vi "Programa Principal.vi"() -> ()   [LabVIEW 2017]
uses:
  <vilib>/Instr/_visa.llb/Select Event Type.ctl
  <vilib>/addons/_office/_exclsub.llb/font.ctl
  <vilib>/Utility/NIReport.llb/Append Report Text (str wrap).vi
  <vilib>/Utility/NIReport.llb/NI_report.lvclass
  <vilib>/addons/_office/NI_ReportGenerationToolkit.lvlib
  <vilib>/Utility/NIReport.llb/Word/NI_Word.lvclass
panel:
  in  "report file path":path
  in  "Guardar":bool
  in  "COMENTARIO":string
  in  "Prac5":bool
  in  "stop 2":bool
  out "Byte recibido":u16
  out "Byte enviado":u32
  out "Datos recibidos":u8[](array[numeric])
  in  "VISA resource name":refnum<visa-resource-name>
  out "Grafica":dbl(graph)
  out "O4":bool
  out "O5":bool
  out "O6":bool
  out "O7":bool
  out "O8":bool
  in  "S4":bool
  in  "S5":bool
  in  "S6":bool
  in  "S7":bool
  in  "S8":bool
  out "Tiempo de Muestreo (ms)":dbl format="%#_5g"
  in  "Semi. Aut.":bool
  in  "Aut.":bool
  out "Manual 2":bool caption="Manual"
  in  "Manual":bool
  out "Automatico 2":bool
  out "Sem.Aut.":bool
  out "Emergencia 2":bool caption="Manual"
  in  "Emergencia":bool
  in  "stop":bool
  in  "Prac4":bool
  in  "Base de Datos":bool
  # "TABLERO DE COMUNICACION"
  # "TABLERO DE CONTRLOL"
  # "ON"
  # "OFF"
  # "LABORATORIO DE MATERIALES"
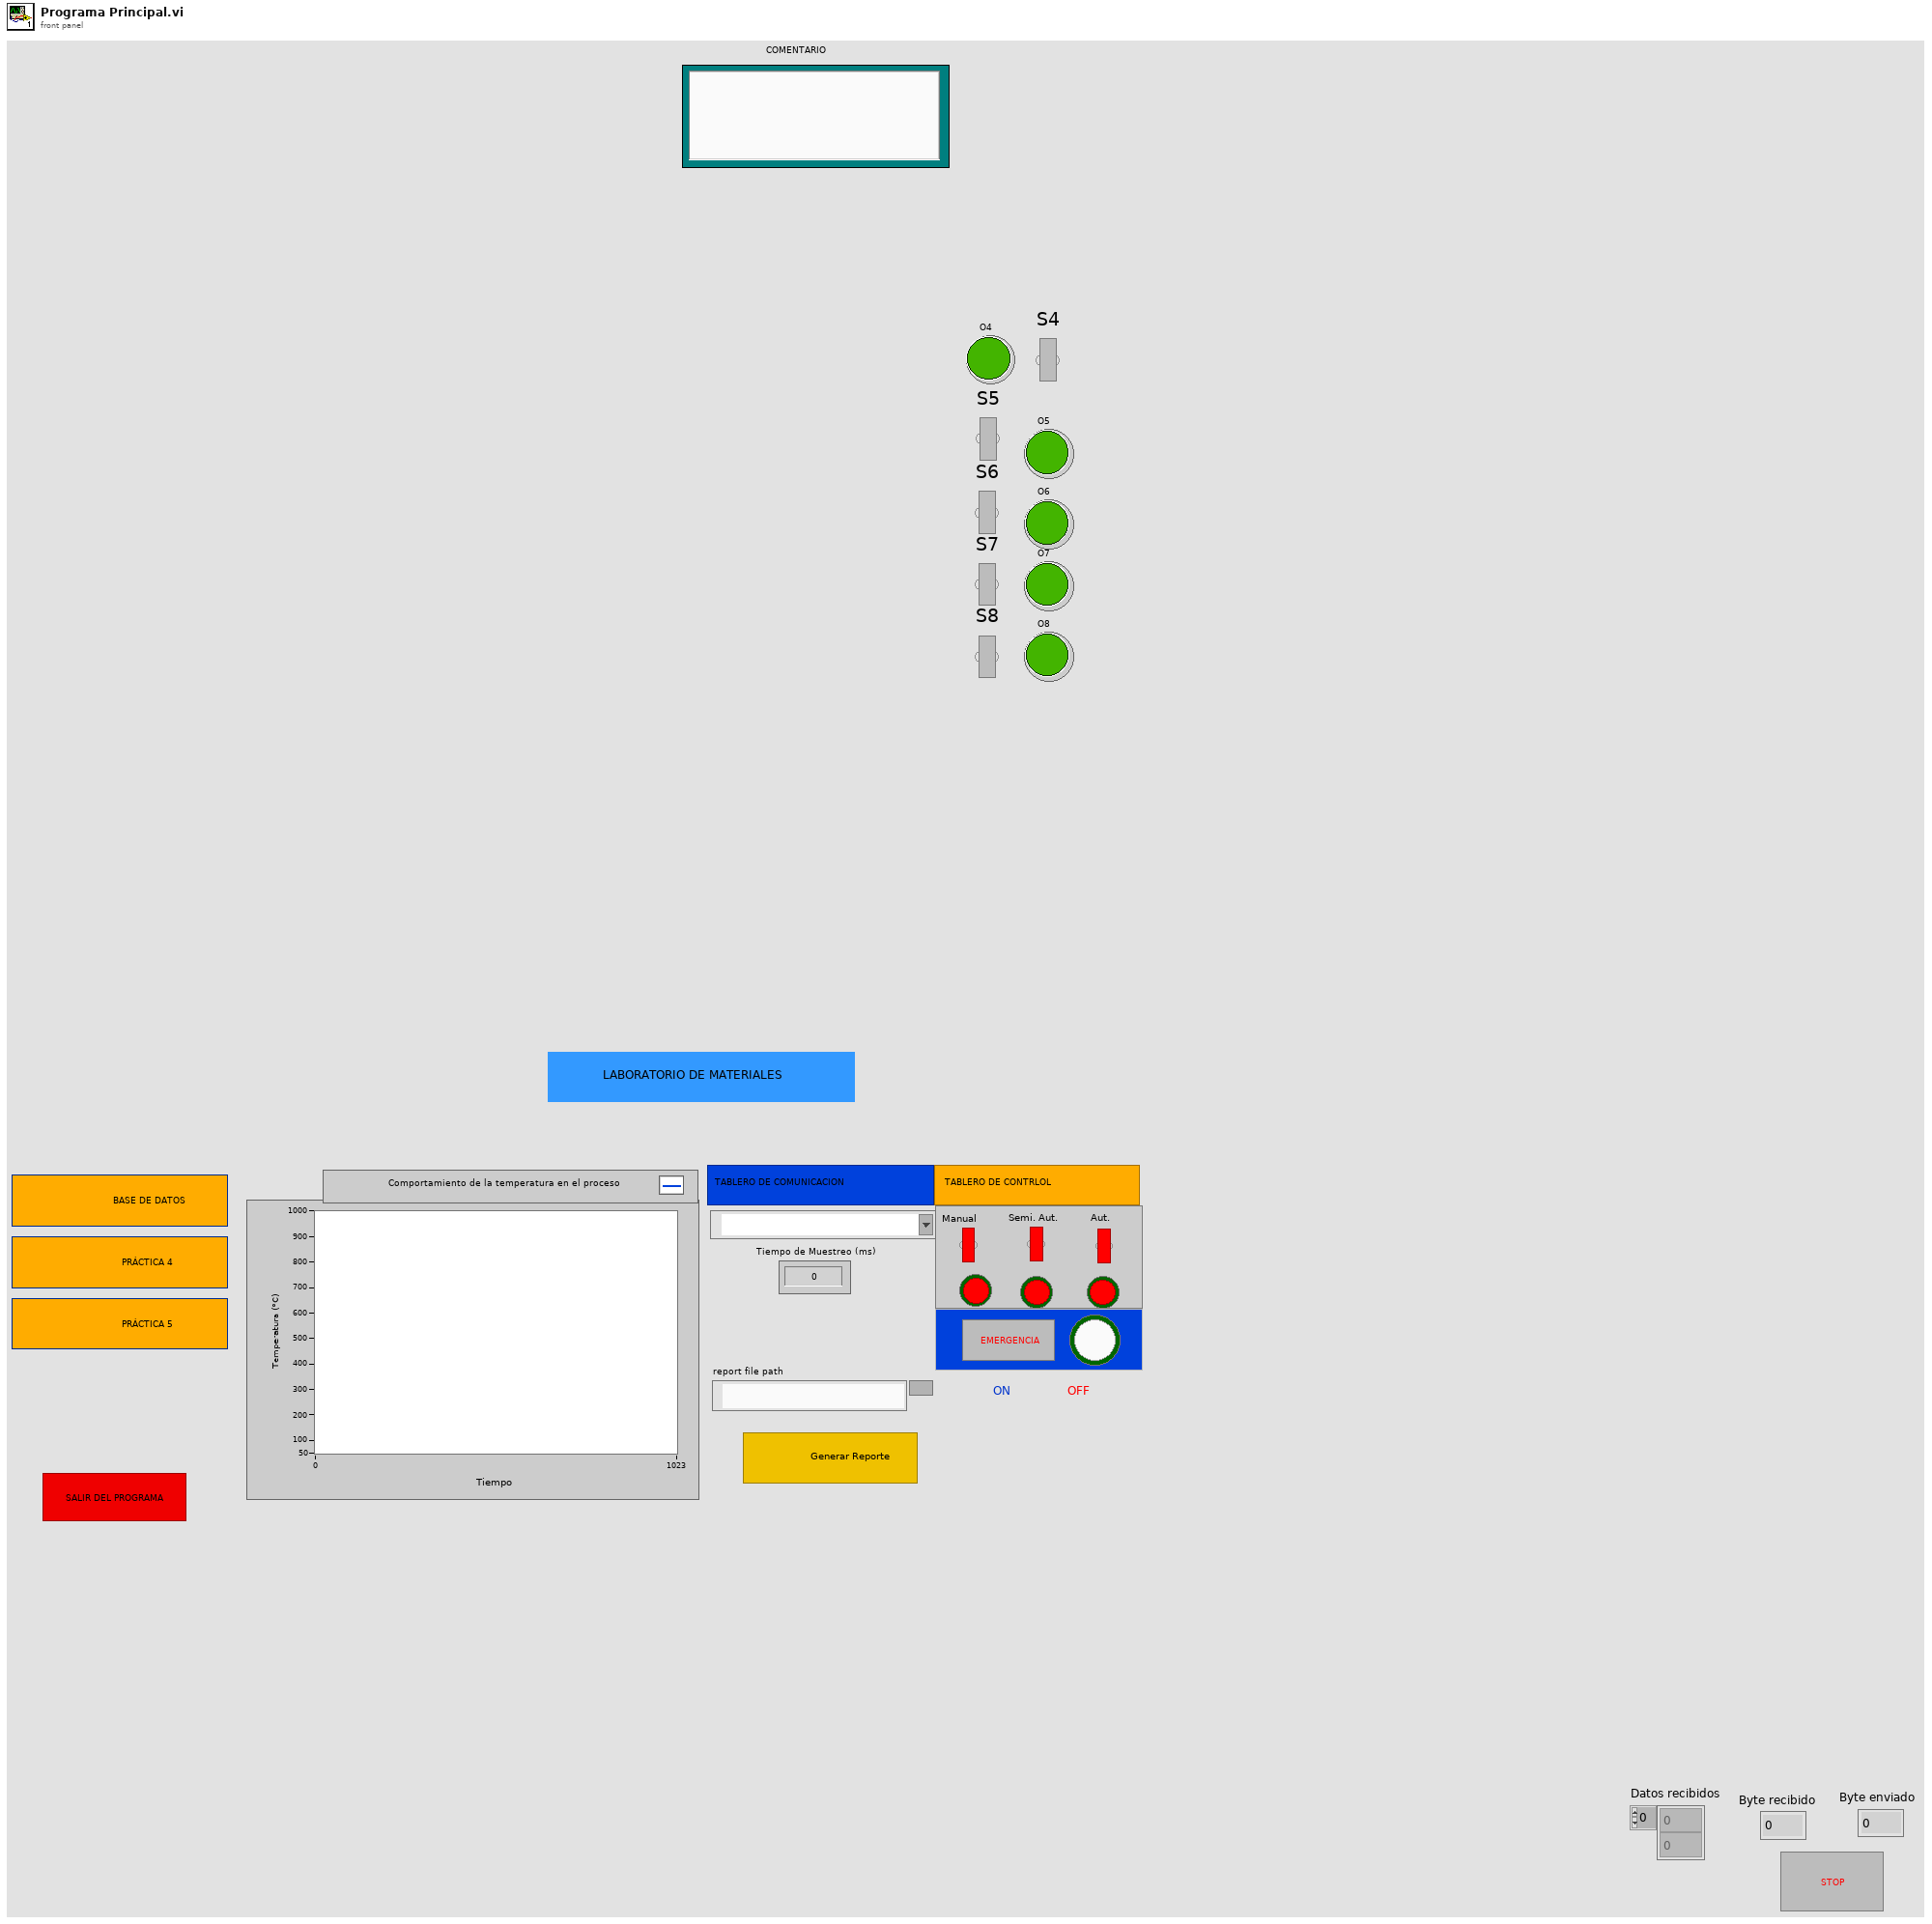
[diagram p1: front panel]
types:
  T1 = cluster{"Charset (-1)":i16, "Weight (-1)":i16, "Name":string, "Size":string}
  T2 = typedef "NI_ReportGenerationToolkit.lvlib/font.ctl" = cluster{"font name":string, "font size":dbl, "bold":u16, "italic":u16, "underline":u16, "strike through":u16, "font color":u32}
  T3 = enum16{"Standard Report", "HTML", "Word", "Excel"}
  T4 = typedef "Select Event Type.ctl" = u32
  T5 = cluster{bool, bool, bool, "S4":bool, "S5":bool, "S6":bool, "S7":bool, "S8":bool}
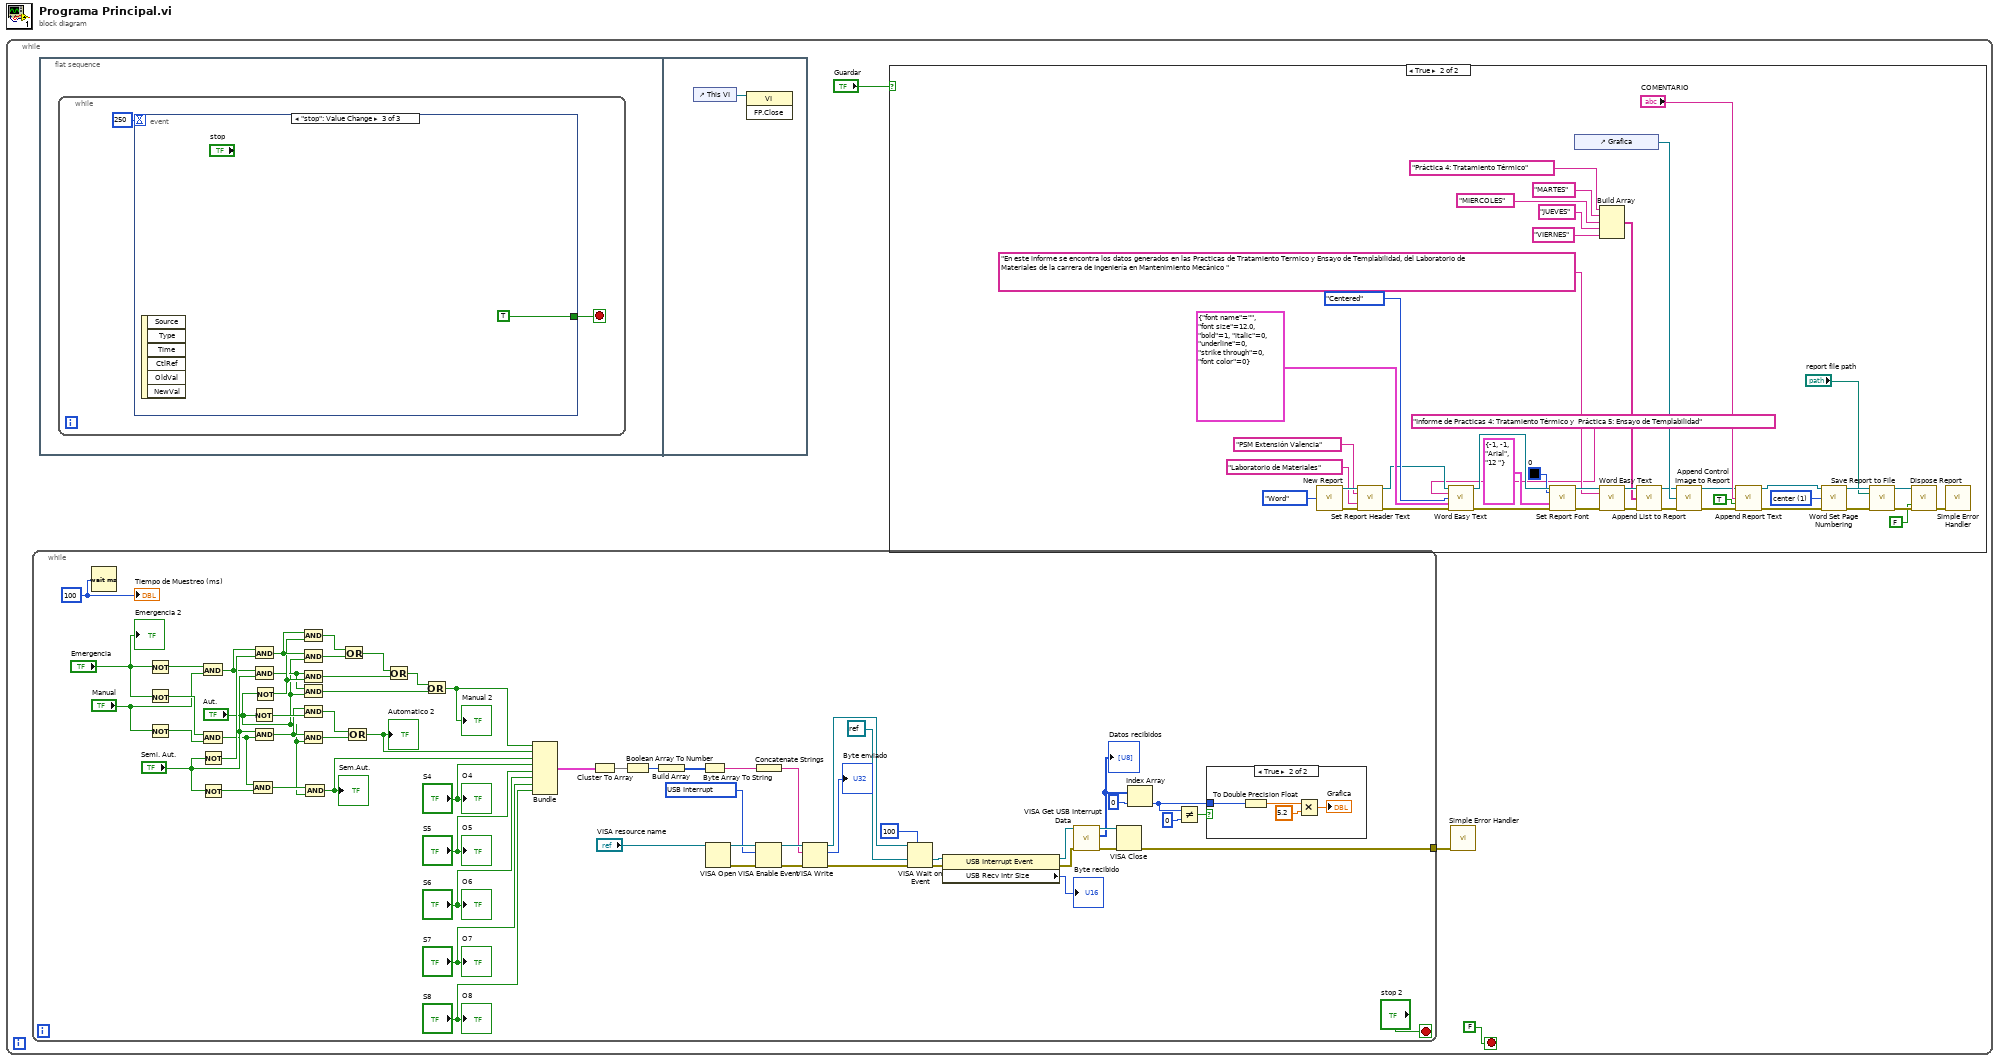
[diagram p0: block diagram]
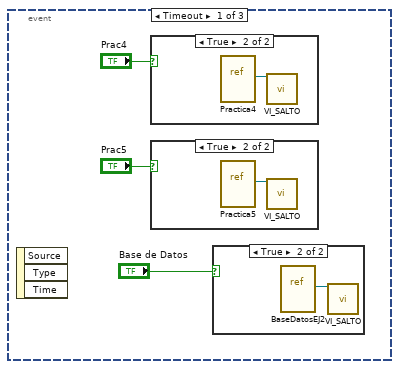
[diagram p4: hidden frame]
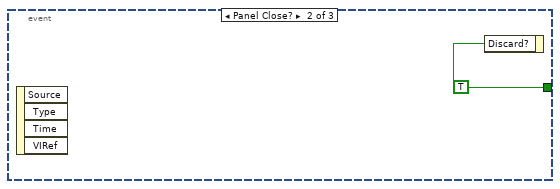
[diagram p8: hidden frame]
diagram:
  n1 = while {
    stop <- FALSE stop-if-true
    n2 = while {
      tunnel: [w100] -> w2
      stop <- "stop 2" stop-if-true
      w82 = u32 100 ("milliseconds to wait")
      w94 = T4 1073684535 items=["Service Request"=1073684491, "Trigger"=3221168138, "Clear"=1073684493, "VXI Signal"=1073684512, "VXI/VME Interrupt"=3221168161, "VXI/VME Sysfail"=1073684509, "VXI/VME Sysreset"=1073684510, "GPIB CIC"=1073684498, "GPIB Talk"=1073684499, "GPIB Listen"=1073684500, "PXI Interrupt"=1073684514, "Serial Break"=1073684515, "Serial TermChar"=1073684516, "Serial CTS"=1073684521, "Serial DSR"=1073684522, "Serial DCD"=1073684524, "Serial RI"=1073684526, "Serial Character"=1073684533, "USB Interrupt"=1073684535, "All Enabled"=1073709055] ("Event Type")
      n3 = Wait (ms)(milliseconds to wait=w82) -> ()  [unwired: 1 out]
      n4 = Not(x="Emergencia") -> (.not. x?=w73:bool)
      n5 = Not(x="Emergencia") -> (.not. x?=w80:bool)
      n6 = Not(x="Manual") -> (.not. x?=w79:bool)
      n7 = And(x=w73, y="Manual") -> (x .and. y?=w68:bool)
      n8 = And(x=w80, y=w79) -> (x .and. y?=w57:bool)
      n9 = Not(x="Semi. Aut.") -> (.not. x?=w72:bool)
      n10 = Not(x="Semi. Aut.") -> (.not. x?=w78:bool)
      n11 = And(x=w57, y=w78) -> (x .and. y?=w81:bool)
      n12 = Not(x="Aut.") -> (.not. x?=w77:bool)
      n13 = And(x=w68, y=w72) -> (x .and. y?=w70:bool)
      n14 = And(x=w68, y="Semi. Aut.") -> (x .and. y?=w64:bool)
      n15 = And(x="Semi. Aut.", y=w57) -> (x .and. y?=w75:bool)
      n16 = Not(x="Aut.") -> (.not. x?=w67:bool)
      n17 = And(x=w70, y=w67) -> (x .and. y?=w71:bool)
      n18 = And(x=w70, y="Aut.") -> (x .and. y?=w69:bool)
      n19 = And(x=w64, y=w67) -> (x .and. y?=w65:bool)
      n20 = And(x=w64, y="Aut.") -> (x .and. y?=w63:bool)
      n21 = And(x=w75, y=w77) -> (x .and. y?=w76:bool)
      n22 = And(x=w75, y="Aut.") -> (x .and. y?=w74:bool)
      n23 = And(x=w81, y="Aut.") -> (x .and. y?=w55:bool)
      "Sem.Aut." <- w55
      n24 = Or(x=w71, y=w69) -> (x .or. y?=w66:bool)
      n25 = Or(x=w76, y=w74) -> (x .or. y?=w56:bool)
      "Automatico 2" <- w56
      n26 = Or(x=w66, y=w65) -> (x .or. y?=w62:bool)
      n27 = Or(x=w62, y=w63) -> (x .or. y?=w61:bool)
      "Manual 2" <- w61
      n28 = Bundle(w61, w56, w55, "S4"="S4", "S5"="S5", "S6"="S6", "S7"="S7", "S8"="S8") -> (w48:T5)  [unwired: 1 in]
      n29 = Cluster To Array(cluster=w48) -> (array=w47:bool[])
      n30 = Boolean Array To Number(Boolean array=w47) -> (number=w85:u32)
      n31 = Build Array(w85) -> (w84:u32[])
      n32 = Byte Array To String(unsigned byte array=w84) -> (string=w83:string)
      n33 = VISA Open(VISA resource name="VISA resource name") -> (VISA resource name=w98:refnum<visa-resource-name>, error out=w97:errorcluster)  [unwired: 4 in]
      n34 = VISA Enable Event(8:w97, 10:w94, 11:w98) -> (0:w95:errorcluster, 3:w96:refnum<visa-resource-name>)  [unwired: 1 in]
      n35 = Concatenate Strings(w83) -> (w46:string)
      n36 = VISA Write(VISA resource name=w96, write buffer=w46, error in (no error)=w95) -> (VISA resource name out=w109:refnum<visa-resource-name>, return count=→"Byte enviado":u32, error out=w99:errorcluster)
      n37 = VISA Wait on Event(7:u32 100 ("General Settings:Timeout Value"), 8:w99, 9:refnum<visa-resource-name> refnum ("event class (Generic Event)"), 11:w109) -> (0:w108:errorcluster, 1:w92:refnum<visa-resource-name>)  [unwired: 1 in, 2 out]
      n38 = property class="USB Interrupt Event"(reference=w92, error in=w108) -> (reference out=w104:refnum<visa-resource-name>, error out=w105:errorcluster, "USB Recv Intr Size"=→"Byte recibido":u16)
      n39 = call <vilib>:"VISA Get USB Interrupt Data.vi"("error in (no error)"=w105, "VISA USB Intr Event"=w104) -> ("error out"=w101:errorcluster, "data buffer"=w90:u8[], "VISA USB Intr Event out"=w102:refnum<visa-resource-name>)  [unwired: 7 in]
      "Datos recibidos" <- w90
      n40 = VISA Close(VISA resource name=w102, error in (no error)=w101) -> (error out=w100:errorcluster)
      n41 = Index Array(array=w90, index=0) -> (element=w88:u8)
      n42 = Not Equal?(x=w88, y=u8 0) -> (x != y?=w86:bool)
      n43 = case shown="True" w86 {
        tunnel: w88 -> [_ w114]
        frame False {
        }
        frame True {
          n44 = To Double Precision Float(number=w114) -> (double precision float=w113:dbl)
          n45 = Multiply(x=w113, y=5.2) -> (x*y=→"Grafica":dbl)
        }
      }
      "O4" <- "S4"
      "O5" <- "S5"
      "O6" <- "S6"
      "O7" <- "S7"
      "O8" <- "S8"
      "Tiempo de Muestreo (ms)" <- w82
      "Emergencia 2" <- "Emergencia"
    }
    n46 = flat-sequence {
      frame #0 {
        n47 = while {
          stop <- w115 stop-if-true
          n48 = event shown="[2] \"stop\": Value Change" {
            selector: _ -> [_ _ _]
            dyn-events: _ -> [_ _ _]
            timeout: 250 -> [_ _ _]
            tunnel: [_ w123 TRUE ("Discard?")] -> w115
            event Timeout {
              n49 = event-data() -> ()  [unwired: 1 in, 3 out]
              n50 = case shown="True" "Prac4" {
                frame False {
                }
                frame True {
                  n51 = vi-ref "Practica4.vi"() -> (w121:refnum<vi>)
                  n52 = call "VI_SALTO.vi"("reference"=w121) -> ()  [unwired: 15 in]
                }
              }
              n53 = case shown="True" "Prac5" {
                frame False {
                }
                frame True {
                  n54 = vi-ref "Practica5.vi"() -> (w120:refnum<vi>)
                  n55 = call "VI_SALTO.vi"("reference"=w120) -> ()  [unwired: 15 in]
                }
              }
              n56 = case shown="True" "Base de Datos" {
                frame False {
                }
                frame True {
                  n57 = vi-ref "BaseDatosEJ2.vi"() -> (w122:refnum<vi>)
                  n58 = call "VI_SALTO.vi"("reference"=w122) -> ()  [unwired: 15 in]
                }
              }
            }
            event Panel Close? {
              w123 = TRUE ("Discard?")
              n59 = event-data() -> ()  [unwired: 1 in, 4 out]
              n60 = event-data("Discard?"=w123) -> ()  [unwired: 1 in, 1 out]
            }
            event "stop": Value Change {
              n61 = event-data() -> ()  [unwired: 1 in, 6 out]
            }
          }
        }
      }
      frame #1 {
        n62 = control-ref of="This VI"() -> (w125:refnum<vi>)
        n63 = invoke class="VI" method="FP.Close"(reference=w125) -> ()  [unwired: 2 in, 3 out]
      }
    }
    n64 = case shown="True" "Guardar" {
      frame False {
      }
      frame True {
        w12 = u16 1 items=["left", "center", "right"] ("alignment (right)")
        n65 = call <vilib>:"New Report.vi"("report type"=T3."Word") -> ("report out"=w43:refnum<class "NI_report.lvclass">, "error out"=w44:errorcluster)  [unwired: 13 in]
        n66 = call-dynamic "Set Report Header Text.vi"("report in"=w43, "left header text"="PSM Extensión Valencia", "right header text"="Laboratorio de Materiales", "error in (no error)"=w44) -> ("report out"=w6:refnum<class "NI_report.lvclass">, "error out"=w7:errorcluster)  [unwired: 10 in]
        n67 = call <vilib>:"Word Easy Text.vi"("report in"=w6, "text"="Informe de Practicas 4: Tratamiento Térmico y  Práctica 5: Ensayo de Templabilidad", "alignment (left)"=enum16{"Left", "Centered", "Right", "Justify"}."Centered", "font"=T2 {"font name"="", "font size"=12.0, "bold"=1, "italic"=0, "underline"=0, "strike through"=0, "font color"=0}, "error in (no error)"=w7) -> ("report out"=w35:refnum<class "NI_report.lvclass">, "error out"=w36:errorcluster)  [unwired: 8 in, 1 out]
        n68 = call-dynamic "Set Report Font.vi"("report in"=w35, "text color (unchanged)"=u32 0, "font settings"=T1 {"Charset (-1)"=-1, "Weight (-1)"=-1, "Name"="Arial", "Size"="12 "}, "error in (no error)"=w36) -> ("report out"=w37:refnum<class "NI_report.lvclass">, "error out"=w38:errorcluster)  [unwired: 9 in, 1 out]
        n69 = control-ref of="Grafica"() -> (w23:refnum<vi>)
        n70 = Build Array("Práctica 4: Tratamiento Térmico", "MARTES", "MIERCOLES", "JUEVES", "VIERNES") -> (w29:string[])
        n71 = call <vilib>:"Word Easy Text.vi"("report in"=w37, "text"="En este informe se encontra los datos generados en las Practicas de Tratamiento Termico y Ensayo de Templabilidad, del Laboratorio de Materiales de la carrera de Ingeniería en Mantenimiento Mecánico ", "error in (no error)"=w38) -> ("report out"=w31:refnum<class "NI_report.lvclass">, "error out"=w32:errorcluster)  [unwired: 10 in, 1 out]
        n72 = call-dynamic "Append List to Report.vi"("report in"=w31, "list elements"=w29, "error in (no error)"=w32) -> ("report out"=w22:refnum<class "NI_report.lvclass">, "error out"=w21:errorcluster)  [unwired: 9 in, 2 out]
        n73 = call-dynamic "Append Control Image to Report.vi"("report in"=w22, "ctrl reference"=w23, "error in (no error)"=w21) -> ("report out"=w18:refnum<class "NI_report.lvclass">, "error out"=w19:errorcluster)  [unwired: 9 in, 2 out]
        n74 = call-poly <vilib>:"Append Report Text.vi"("report in"=w18, "text"="COMENTARIO", "append on new line? (F)"=TRUE, "error in (no error)"=w19) -> ("report out"=w13:refnum<class "NI_report.lvclass">, "error out"=w14:errorcluster)  [unwired: 8 in, 2 out]
        n75 = call <vilib>:"Word Set Page Numbering.vi"("report in"=w13, "alignment (right)"=w12, "error in (no error)"=w14) -> ("report out"=w16:refnum<class "NI_report.lvclass">, "error out"=w15:errorcluster)  [unwired: 11 in]
        n76 = call-dynamic "Save Report to File.vi"("report in"=w16, "report file path"="report file path", "error in (no error)"=w15) -> ("report out"=w9:refnum<class "NI_report.lvclass">, "error out"=w11:errorcluster)  [unwired: 11 in]
        n77 = call-dynamic "Dispose Report.vi"("report in"=w9, "error in (no error)"=w11, "close report? (T)"=FALSE) -> ("error out"=w10:errorcluster)  [unwired: 12 in]
        n78 = call <vilib>:"Simple Error Handler.vi"("error in (no error)"=w10) -> ()  [unwired: 4 in, 5 out]
      }
    }
    n79 = call <vilib>:"Simple Error Handler.vi"("error in (no error)"=w2) -> ()  [unwired: 4 in, 5 out]
  }
